vi "MAT Save Matrix.vi"(0 "Ref Num":refnum<file>, 1 "DBL":dbl[][](array[numeric]) format="%.2f", 2 "SGL":sgl[][](array[numeric]) format="%.2f", 3 "I32":i32[][](array[numeric]), 4 "I16":i16[][](array[numeric]), 5 "error in":errorcluster, 6 "Matrix Name":string, 7 "U16":u16[][](array[numeric]), 9 "U8":u8[][](array[numeric]), 10 "STR":string[](array[string]), 11 "CDB":cdb[][](array[numeric]) format="%.2f", 13 "CSG":csg[][](array[numeric]) format="%.2f") -> (14 "Dup Ref Num":refnum<file>, 19 "error out":errorcluster)   [LabVIEW 2020, in "GOLPI library.lvlib"]
doc: "\"Save to MAT\" saves a 2D array of numbers or a 1D array of strings to MATLAB file. It works only with LabVIEW for Windows. All data types, described in MATLAB/External Interface Guide/Appendix A, are supported, except Sparse Matrices.\n\nAll data inputs should be 2D arrays, except String input which should be a 1D array. Only one data input may contain a non-empty array, otherwise error will be generated (error code -1).\n\nSAVML.LLB is a freeware written by Serge Liberman <liber@us1.channel1.com>."
uses:
  GOLPI library.lvlib
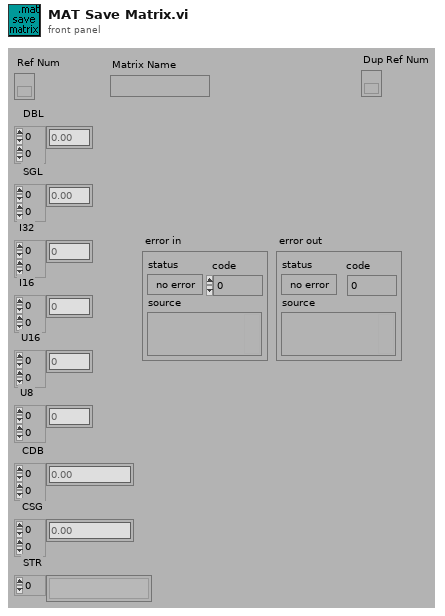
[diagram p1: front panel]
types:
  T1 = enum16{"big-endian, network order", "native, host order", "little-endian"}
  T2 = typedef "GOLPI library.lvlib/MAT Type Representation.ctl" = enum16{"DBL", "SGL", "I32", "I16", "U16", "U8", "CDB", "CSG", "STR"}
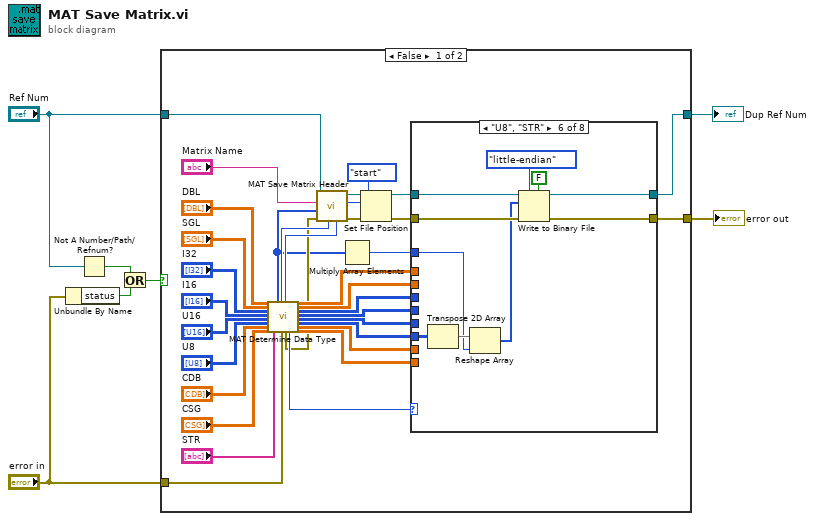
[diagram p0: block diagram]
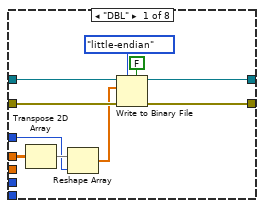
[diagram p2: hidden frame]
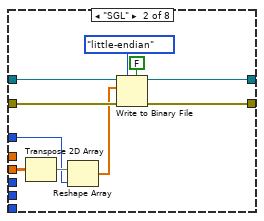
[diagram p3: hidden frame]
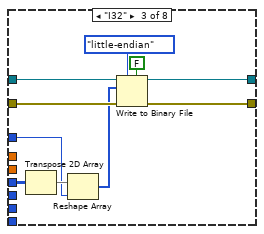
[diagram p4: hidden frame]
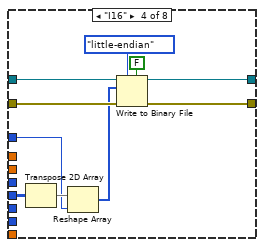
[diagram p5: hidden frame]
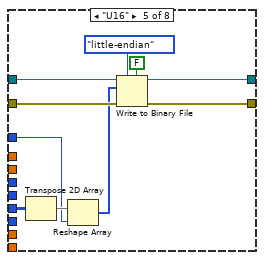
[diagram p6: hidden frame]
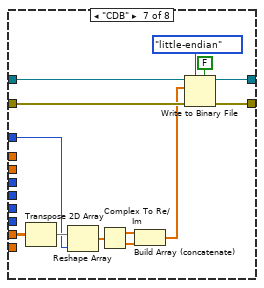
[diagram p7: hidden frame]
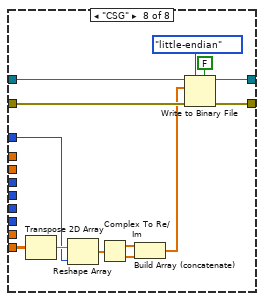
[diagram p8: hidden frame]
diagram:
  n1 = Unbundle By Name("error in") -> ("status"=w4:bool)
  n2 = Not A Number/Path/Refnum?(number/path/refnum="Ref Num") -> (NaN/Path/Refnum?=w2:bool)
  n3 = Or(x=w2, y=w4) -> (x .or. y?=w1:bool)
  n4 = case shown="False" w1 {
    tunnel: [w8 w129] -> w7
    tunnel: "Ref Num" -> [w41 w129]
    tunnel: "error in" -> [w18 w128]
    tunnel: [w40 w128] -> w5
    frame False {
      n5 = call "MAT Determine Data Type.vi"("DBL"="DBL", "SGL"="SGL", "I32"="I32", "I16"="I16", "U16"="U16", "U8"="U8", "CDB"="CDB", "CSG"="CSG", "STR"="STR", "error in (no error)"=w18) -> ("Matrix Size"=w16:i32[], "Rep. Code"=w20:u32, "Real/Complex (0-Real)"=w21:u32, "error out"=w17:errorcluster, "Representation"=w19:T2, "DBL copy"=w29:dbl[][], "SGL copy"=w28:sgl[][], "I32 copy"=w27:i32[][], "I16 copy"=w26:i16[][], "U16 copy"=w25:u16[][], "U8 copy"=w24:u8[][], "CDB copy"=w23:cdb[][], "CSG copy"=w22:csg[][])  [unwired: 5 in]
      n6 = call "MAT Save Matrix Header.vi"("Real/Complex (0-Real)"=w21, "Rep. Code"=w20, "error in (no error)"=w17, "Matrix Size"=w16, "Matrix Name"="Matrix Name", "Ref Num"=w41) -> ("error out"=w14:errorcluster, "offset"=w10:i32, "Dup Ref Num"=w12:refnum<file>)  [unwired: 3 in]
      n7 = Multiply Array Elements(1:w16) -> (0:w15:i32)
      n8 = Set File Position(offset (in bytes) (0)=w10, refnum=w12, from (0:start)=enum16{"start", "end", "current"}."start", error in=w14) -> (refnum out=w11:refnum<file>, error out=w13:errorcluster)
      n9 = case shown="\"U8\", \"STR\"" w19 {
        tunnel: w11 -> [w47 w58 w68 w78 w88 w98 w111 w124]
        tunnel: w29 -> [w51 _ _ _ _ _ _ _]
        tunnel: w28 -> [_ w52 _ _ _ _ _ _]
        tunnel: w27 -> [_ _ w62 _ _ _ _ _]
        tunnel: w26 -> [_ _ _ w72 _ _ _ _]
        tunnel: w25 -> [_ _ _ _ w82 _ _ _]
        tunnel: w24 -> [_ _ _ _ _ w92 _ _]
        tunnel: w23 -> [_ _ _ _ _ _ w106 _]
        tunnel: w22 -> [_ _ _ _ _ _ _ w115]
        tunnel: [w42 w53 w63 w73 w83 w93 w107 w120] -> w8
        tunnel: w13 -> [w48 w59 w69 w79 w89 w99 w112 w125]
        tunnel: [w43 w54 w64 w74 w84 w94 w108 w121] -> w40
        tunnel: w15 -> [w49 w60 w70 w80 w90 w100 w113 w126]
        frame "DBL" {
          n10 = Transpose 2D Array(2D array=w51) -> (transposed array=w50:dbl[][])
          n11 = Reshape Array(w50, w49) -> (w46:dbl[])
          n12 = Write to Binary File(file (use dialog)=w47, data=w46, error in=w48, 5:FALSE ("prepend array or string size? (T)"), 9:T1."little-endian" ("byte order (0:big-endian, network order)")) -> (refnum out=w42:refnum<file>, error out=w43:errorcluster)  [unwired: 1 in, 1 out]
        }
        frame "SGL" {
          n13 = Transpose 2D Array(2D array=w52) -> (transposed array=w61:sgl[][])
          n14 = Reshape Array(w61, w60) -> (w57:sgl[])
          n15 = Write to Binary File(file (use dialog)=w58, data=w57, error in=w59, 5:FALSE ("prepend array or string size? (T)"), 9:T1."little-endian" ("byte order (0:big-endian, network order)")) -> (refnum out=w53:refnum<file>, error out=w54:errorcluster)  [unwired: 1 in, 1 out]
        }
        frame "I32" {
          n16 = Transpose 2D Array(2D array=w62) -> (transposed array=w71:i32[][])
          n17 = Reshape Array(w71, w70) -> (w67:i32[])
          n18 = Write to Binary File(file (use dialog)=w68, data=w67, error in=w69, 5:FALSE ("prepend array or string size? (T)"), 9:T1."little-endian" ("byte order (0:big-endian, network order)")) -> (refnum out=w63:refnum<file>, error out=w64:errorcluster)  [unwired: 1 in, 1 out]
        }
        frame "I16" {
          n19 = Transpose 2D Array(2D array=w72) -> (transposed array=w81:i16[][])
          n20 = Reshape Array(w81, w80) -> (w77:i16[])
          n21 = Write to Binary File(file (use dialog)=w78, data=w77, error in=w79, 5:FALSE ("prepend array or string size? (T)"), 9:T1."little-endian" ("byte order (0:big-endian, network order)")) -> (refnum out=w73:refnum<file>, error out=w74:errorcluster)  [unwired: 1 in, 1 out]
        }
        frame "U16" {
          n22 = Transpose 2D Array(2D array=w82) -> (transposed array=w91:u16[][])
          n23 = Reshape Array(w91, w90) -> (w87:u16[])
          n24 = Write to Binary File(file (use dialog)=w88, data=w87, error in=w89, 5:FALSE ("prepend array or string size? (T)"), 9:T1."little-endian" ("byte order (0:big-endian, network order)")) -> (refnum out=w83:refnum<file>, error out=w84:errorcluster)  [unwired: 1 in, 1 out]
        }
        frame "U8", "STR" {
          n25 = Transpose 2D Array(2D array=w92) -> (transposed array=w101:u8[][])
          n26 = Reshape Array(w101, w100) -> (w97:u8[])
          n27 = Write to Binary File(file (use dialog)=w98, data=w97, error in=w99, 5:FALSE ("prepend array or string size? (T)"), 9:T1."little-endian" ("byte order (0:big-endian, network order)")) -> (refnum out=w93:refnum<file>, error out=w94:errorcluster)  [unwired: 1 in, 1 out]
        }
        frame "CDB" {
          n28 = Transpose 2D Array(2D array=w106) -> (transposed array=w114:cdb[][])
          n29 = Reshape Array(w114, w113) -> (w105:cdb[])
          n30 = Complex To Re/Im(x + iy=w105) -> (x=w104:dbl[], y=w103:dbl[])
          n31 = Build Array (concatenate)(w104, w103) -> (w102:dbl[])
          n32 = Write to Binary File(file (use dialog)=w111, data=w102, error in=w112, 5:FALSE ("prepend array or string size? (T)"), 9:T1."little-endian" ("byte order (0:big-endian, network order)")) -> (refnum out=w107:refnum<file>, error out=w108:errorcluster)  [unwired: 1 in, 1 out]
        }
        frame "CSG" {
          n33 = Transpose 2D Array(2D array=w115) -> (transposed array=w127:csg[][])
          n34 = Reshape Array(w127, w126) -> (w119:csg[])
          n35 = Complex To Re/Im(x + iy=w119) -> (x=w118:sgl[], y=w117:sgl[])
          n36 = Build Array (concatenate)(w118, w117) -> (w116:sgl[])
          n37 = Write to Binary File(file (use dialog)=w124, data=w116, error in=w125, 5:FALSE ("prepend array or string size? (T)"), 9:T1."little-endian" ("byte order (0:big-endian, network order)")) -> (refnum out=w120:refnum<file>, error out=w121:errorcluster)  [unwired: 1 in, 1 out]
        }
      }
    }
    frame True {
    }
  }
  "error out" <- w5
  "Dup Ref Num" <- w7
